vi "Tester Present Command.vi"(4 "Numeric Request":u32, 5 "ID Response":string="18DAF255", 6 "ID Request":string="18DA55F2", 7 "Read":refnum<k21>, 8 "Write":refnum<k21>) -> (0 "Read out":refnum<k21>, 1 "Write out":refnum<k21>, 2 "ID String 2":string, 3 "Data String 2":string)   [LabVIEW 2023]
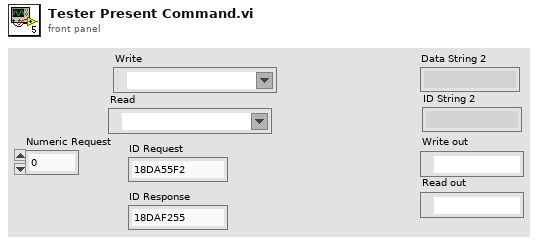
[diagram p1: front panel]
types:
  T1 = typedef "XNET Frame CAN.ctl" = cluster{"timestamp":timestamp, "payload":u8[], "identifier":u32, "type":T2, "extended?":bool, "echo?":bool}
  T2 = typedef "XNET Frame Type CAN.ctl" = u8
  T3 = cluster{"data[0]":T1, "data[1]":T1, "data[2]":T1, "data[3]":T1, "data[4]":T1, "data[5]":T1, "data[6]":T1, "data[7]":T1, "data[8]":T1}
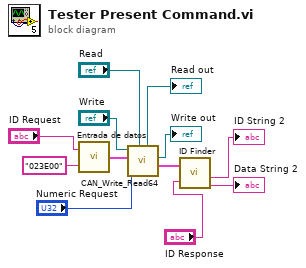
[diagram p0: block diagram]
diagram:
  n1 = call "Entrada de datos.vi"("string"="023E00" ("string 2"), "ID"="ID Request") -> ("CAN frame"=w6:T1)
  n2 = call "CAN_Write_Read64.vi"("Read In"="Read", "Numeric Request"="Numeric Request", "CAN frame"=w6, "Write In"="Write") -> ("cluster"=w5:T3, "Write Out"=→"Write out":refnum<k21>, "Read Out"=→"Read out":refnum<k21>)  [unwired: 1 in, 2 out]
  n3 = call "ID Finder.vi"("cluster"=w5, "ID ESPERADO STRING"="ID Response") -> ("ID String"=→"ID String 2":string, "Data String"=→"Data String 2":string)  [unwired: 4 out]
